vi "write_subtable_key_string.vi"(7 "subtables":string[](array[string]), 8 "error in (no error)":errorcluster, 9 "Item":refnum<class "Item.lvclass">, 10 "subkeys":string[](array[string]), 11 "toml in":refnum<class "toml.lvclass">) -> (0 "error out":errorcluster, 3 "toml out":refnum<class "toml.lvclass">)   [LabVIEW 2020, in "toml.lvclass"]
uses:
  toml.lvclass
  Item/Item.lvclass
  toml.lvclass/toml.ctl
  Doc/Doc.lvclass
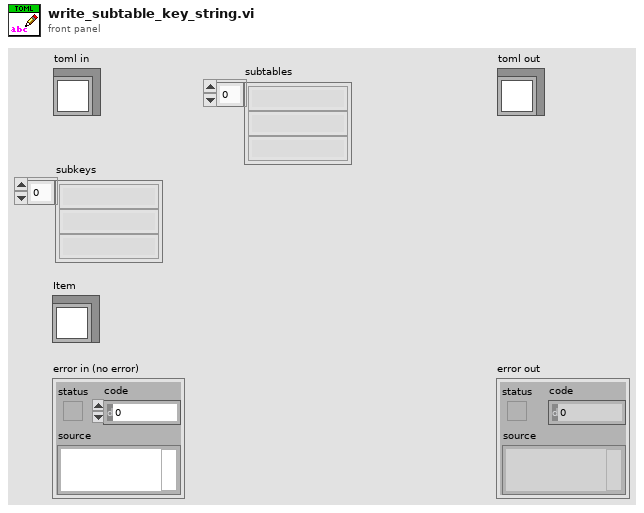
[diagram p1: front panel]
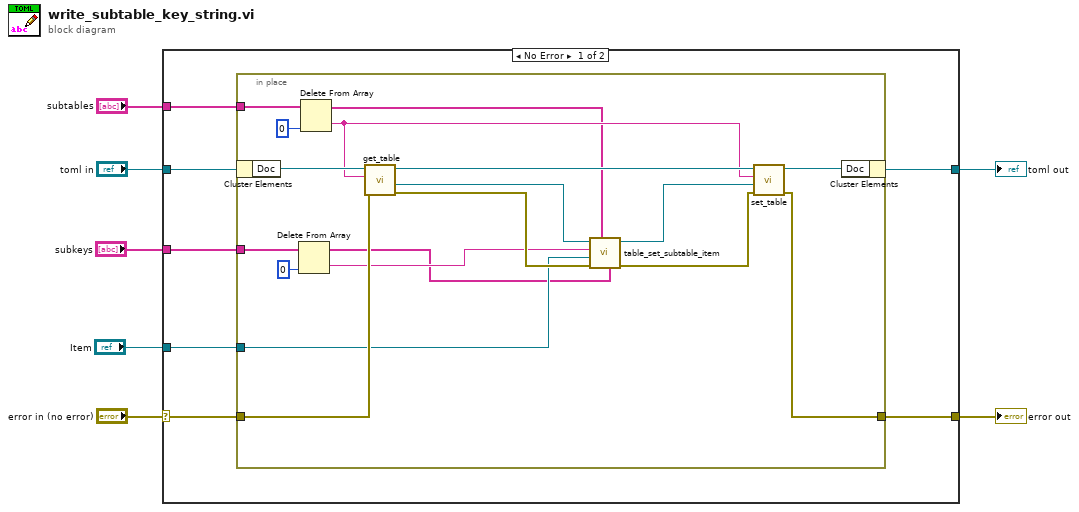
[diagram p0: block diagram]
diagram:
  n1 = case shown="No Error" "error in (no error)" {
    selector: "error in (no error)" -> [w8 w34]
    tunnel: [w9 w34] -> w6
    tunnel: [w13 w33] -> w4
    tunnel: "toml in" -> [w14 w33]
    tunnel: "subtables" -> [w12 _]
    tunnel: "subkeys" -> [w11 _]
    tunnel: "Item" -> [w10 _]
    frame No Error {
      n2 = in-place {
        in-place-border: w12 -> [w23]
        in-place-border: w11 -> [w19]
        in-place-border: w10 -> [w18]
        in-place-border: [w26] -> w9
        in-place-border: w8 -> [w25]
        n3 = in-place-cluster #1(w14) -> ("Doc"=w29:refnum<class "Doc.lvclass">)
        n4 = Delete From Array(array=w19, index=0) -> (deleted portion=w16:string, array with subset deleted=w15:string[])  [unwired: 1 in]
        n5 = Delete From Array(array=w23, index=0) -> (deleted portion=w22:string, array with subset deleted=w20:string[])  [unwired: 1 in]
        n6 = call "get_table.vi"("error in (no error)"=w25, "table_name"=w22, "Doc in"=w29) -> ("error out"=w21:errorcluster, "Table"=w32:refnum<class "Table.lvclass">, "Doc out"=w31:refnum<class "Doc.lvclass">)  [unwired: 5 in, 1 out]
        n7 = call "table_set_subtable_item.vi"("subkeys"=w15, "subtables"=w20, "error in (no error)"=w21, "item (value)"=w18, "key"=w16, "Table in"=w32) -> ("error out"=w27:errorcluster, "Table out"=w30:refnum<class "Table.lvclass">)  [unwired: 4 in]
        n8 = call "set_table.vi"("error in (no error)"=w27, "Table"=w30, "table_name"=w22, "Doc in"=w31) -> ("error out"=w26:errorcluster, "Doc out"=w28:refnum<class "Doc.lvclass">)  [unwired: 6 in]
        n9 = in-place-cluster #1("Doc"=w28) -> (w13:refnum<class "toml.lvclass">)
      }
    }
    frame Error {
    }
  }
  "error out" <- w6
  "toml out" <- w4
